vi "Read Command Processor Status.vi"(8 "error in (no error)":errorcluster, 11 "Command Processor in":refnum<class "Command Processor.lvclass">) -> (0 "error out":errorcluster, 2 "Command Processor Status":T1, 3 "Command Processor out":refnum<class "Command Processor.lvclass">)   [LabVIEW 2013, in "Command Processor.lvlib" / "Command Processor.lvclass"]
uses:
  Command Processor.lvclass
  Command Processor Status.ctl
  Current Previous State Status.ctl
  State Status.ctl
  Command/Command Status.ctl
  Command/State Status.ctl
  Command Processor.lvclass/Command Processor.ctl
  Command/Command.lvclass
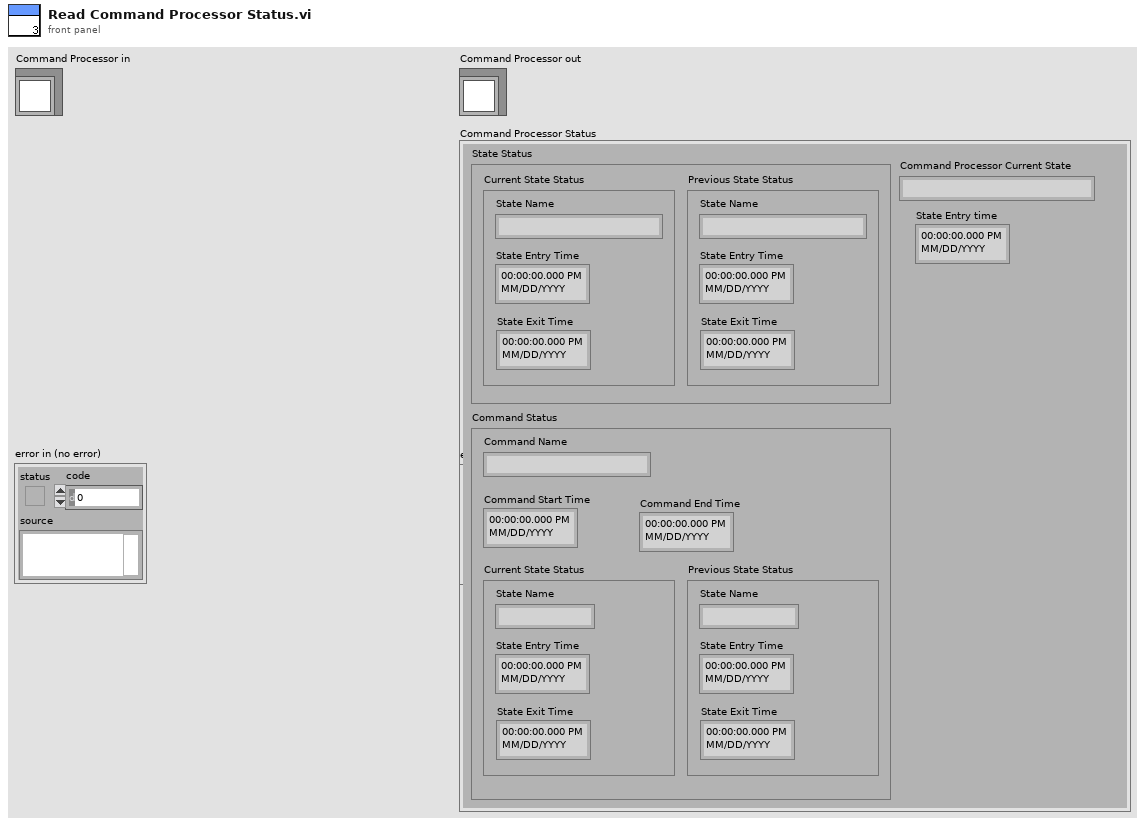
[diagram p1: front panel]
types:
  T1 = typedef "Command Processor.lvlib/Command Processor.lvclass/Command Processor Status.ctl" = cluster{"State Entry time":timestamp, "State Status":T2, "Command Processor Current State":string, "Command Status":T4}
  T2 = typedef "Current Previous State Status.ctl" = cluster{"Current State Status":T3, "Previous State Status":T3}
  T3 = typedef "State Status.ctl" = cluster{"State Name":string, "State Entry Time":timestamp, "State Exit Time":timestamp}
  T4 = typedef "Command Processor.lvlib/Command.lvlib/Command.lvclass/Command Status.ctl" = cluster{"Command Name":string, "Current State Status":T5, "Command Start Time":timestamp, "Command End Time":timestamp, "Previous State Status":T5}
  T5 = typedef "Command Processor.lvlib/Command.lvlib/Command.lvclass/State Status.ctl" = cluster{"State Name":string, "State Entry Time":timestamp, "State Exit Time":timestamp}
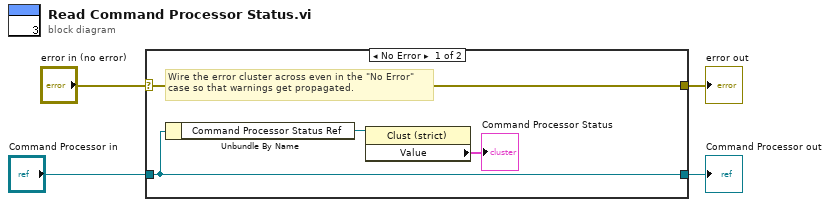
[diagram p0: block diagram]
diagram:
  n1 = case shown="No Error" "error in (no error)" {
    selector: "error in (no error)" -> [w8 w10]
    tunnel: [w8 w10] -> w3
    tunnel: [w7 w9] -> w1
    tunnel: "Command Processor in" -> [w7 w9]
    frame No Error {
      # "Wire the error cluster across even in the \"No Error\"\ncase so that warnings get propagated."
      n2 = Unbundle By Name(w7) -> ("Command Processor Status Ref"=w6:refnum<vi>)
      n3 = property class="Clust (strict)"(reference=w6) -> ("Value"=→"Command Processor Status":T1)  [unwired: 1 in, 2 out]
    }
    frame Error {
    }
  }
  "error out" <- w3
  "Command Processor out" <- w1
